vi "Read Attributes.vi"(11 "Stop Test Msg":refnum<class "Stop Test Msg.lvclass">) -> (2 "Payload":cluster{"Stop Test":bool})   [LabVIEW 2017, in "User Interface.lvlib" / "Stop Test Msg.lvclass"]
uses:
  Stop Test Msg.lvclass
  Stop Test Msg.lvclass/Stop Test Msg.ctl
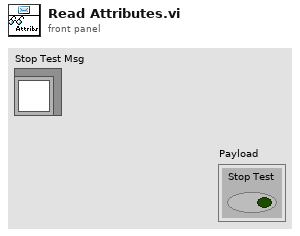
[diagram p1: front panel]
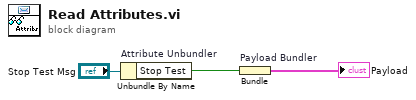
[diagram p0: block diagram]
diagram:
  n1 = Unbundle By Name "Attribute Unbundler"("Stop Test Msg") -> ("Stop Test"=w1:bool)
  n2 = Bundle "Payload Bundler"("Stop Test"=w1) -> (→"Payload":cluster{"Stop Test":bool})  [unwired: 1 in]
